vi "N_Simu_Temp.vi"(9 "Lmax":dbl, 10 "Lmin":dbl, 11 "Numeric":i32) -> (3 "Array":dbl[](array[numeric]))   [LabVIEW 2020]
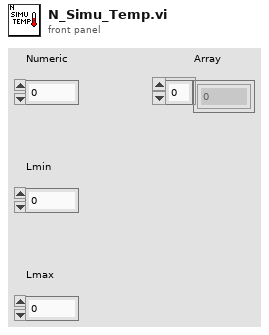
[diagram p1: front panel]
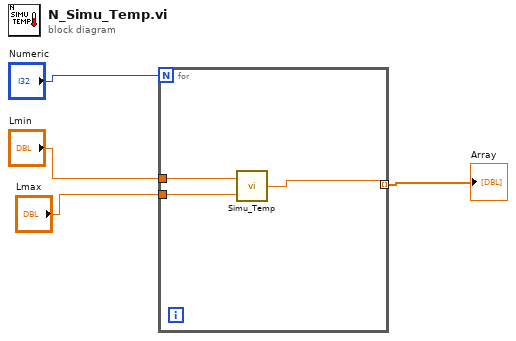
[diagram p0: block diagram]
diagram:
  n1 = for {
    N: "Numeric" -> [_]
    tunnel: "Lmin" -> [w7]
    tunnel: "Lmax" -> [w6]
    tunnel: [w5] -> w4 mode=indexing
    n2 = call "Simu_Temp.vi"("Lmax"=w6, "Lmin"=w7) -> ("Numeric"=w5:dbl)
  }
  "Array" <- w4
